vi "ClientForSingleDeviceDServer_01.vi"() -> ()   [LabVIEW 2014, in "examples.lvlib"]
uses:
  vis/tango_vi.llb/avToShortImage.vi
  vis/tango_vi.llb/avToLongSpectrum.vi
  vis/tango_vi.llb/avToDoubleScalar.vi
  vis/tango_vi.llb/avToStringScalarAv.vi
  examples.lvlib
  vis/tango_vi.llb/tango.lvlib
panel:
  out "timestamp":string
  out "?":string
  out "attribute name":string
  out "quality":string
  out "?":i16[][](graph)
  out "value":dbl(graph)
  out "?":i32[](graph)
  out "success":bool=TRUE
  in  "<TangoTest> device name":string="labview/device/1"
  in  "Attribute names":string[](array[string])=["devDoubleScalar", "devLongSpectrum", "devShortImage", "devStringScalar"]
  # "TANGO  Binding for LabVIEW - LabVIEW DServer Client Example"
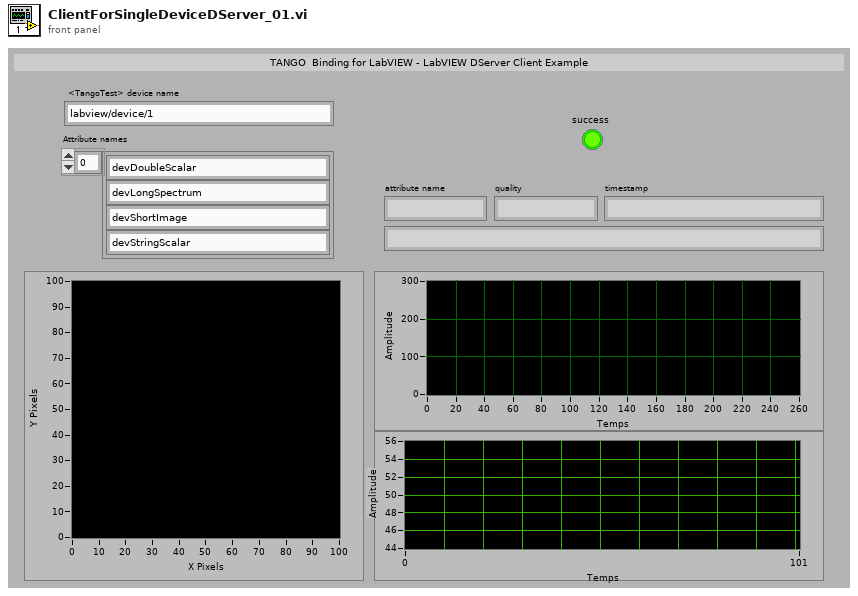
[diagram p1: front panel]
types:
  T1 = typedef "tango.lvlib/_AttributeValue_t.ctl" = cluster{"device name":string, "attribute name":string, "quality value":T2, "quality string":string, "timestamp":dbl, "dim. x":i32, "dim. y":i32, "value":u8[], "error code":i32, "error stack":string[], "data type":T3}
  T2 = typedef "tango.lvlib/_AttributeQuality_t.ctl" = enum16{"VALID", "INVALID", "ALARM", "CHANGING", "UNKNOWN_QUALITY"}
  T3 = typedef "tango.lvlib/_AttributeDataType_t.ctl" = enum16{"STATE_SCA", "STATE_SPE", "STATE_IMG", "STRING_SCA", "STRING_SPE", "STRING_IMG", "BOOL_SCA", "BOOL_SPE", "BOOL_IMG", "UCHAR_SCA", "UCHAR_SPE", "UCHAR_IMG", "SHORT_SCA", "SHORT_SPE", "SHORT_IMG", "USHORT_SCA", "USHORT_SPE", "USHORT_IMG", "LONG_SCA", "LONG_SPE", "LONG_IMG", "ULONG_SCA", "ULONG_SPE", "ULONG_IMG", "LONG64_SCA", "LONG64_SPE", "LONG64_IMG", "ULONG64_SCA", "ULONG64_SPE", "ULONG64_IMG", "FLOAT_SCA", "FLOAT_SPE", "FLOAT_IMG", "DOUBLE_SCA", "DOUBLE_SPE", "DOUBLE_IMG", "ENUM_SCA", "UNKNOWN_DATA_TYPE"}
  T4 = cluster{"device name":string, "attribute name":string, "quality value":i16, "quality string":string, "timestamp":dbl, "dim. x":i32, "dim. y":i32, "value_out":string, "setpoint":string, "error code":i32, "error stack":string[], "data type":u16}
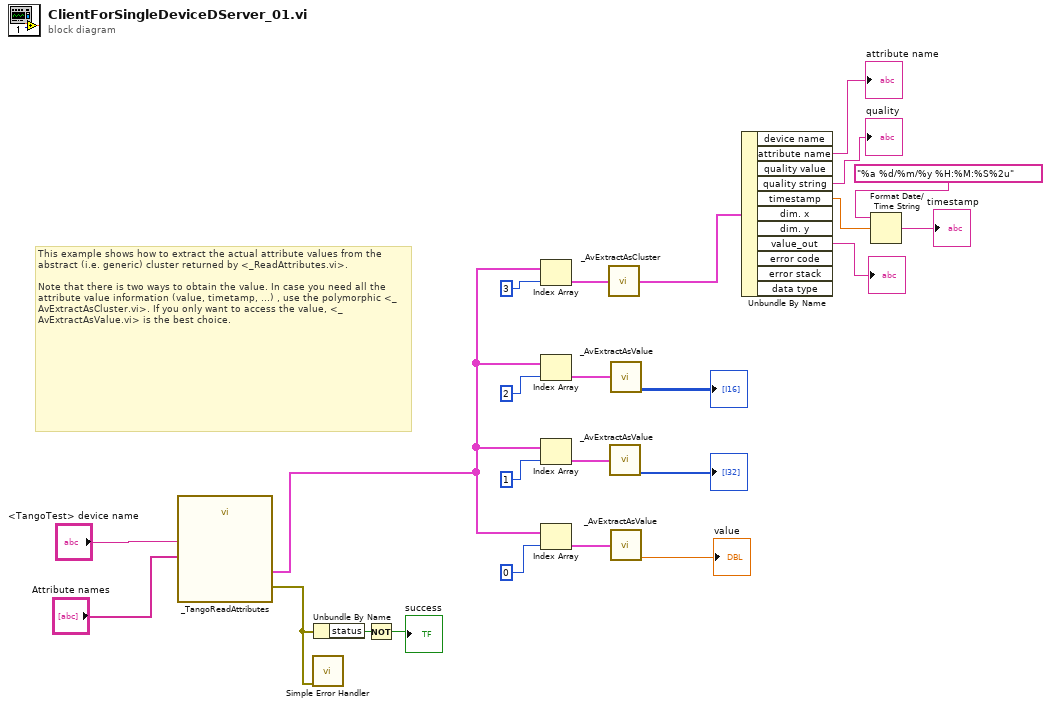
[diagram p0: block diagram]
diagram:
  # "This example shows how to extract the actual attribute values from the abstract (i.e. generic) cluster returned by <_ReadAttributes.vi>. \n\nNote that there is two ways to obtain the value. In case you need all the attribute value information (value, timetamp, ...) , use the polymorphic <_AvExtractAsCluster.vi>. If you only want to access the value, <_AvExtractAsValue.vi> is the best choice."
  n1 = call "_TangoReadAttributes.vi"("attribute names"="Attribute names", "device name"="<TangoTest> device name") -> ("error out"=w2:errorcluster, "attribute values"=w24:T1[])  [unwired: 1 in]
  n2 = call <vilib>:"Simple Error Handler.vi"("error in (no error)"=w2) -> ()  [unwired: 4 in, 5 out]
  n3 = Unbundle By Name(w2) -> ("status"=w3:bool)
  n4 = Not(x=w3) -> (.not. x?=→"success":bool)
  n5 = Index Array(array=w24, index=3 ("indice")) -> (element=w8:T1)
  n6 = Index Array(array=w24, index=2 ("indice")) -> (element=w7:T1)
  n7 = Index Array(array=w24, index=1 ("indice")) -> (element=w6:T1)
  n8 = Index Array(array=w24, index=0 ("indice")) -> (element=w5:T1)
  n9 = call-poly "_AvExtractAsCluster.vi"("attribute value"=w8) -> ("av"=w15:T4)
  n10 = call-poly "_AvExtractAsValue.vi"("attribute value"=w6) -> ("value"=→"?":i32[])  [unwired: 4 out]
  n11 = call-poly "_AvExtractAsValue.vi"("attribute value"=w7) -> ("value"=→"?":i16[][])  [unwired: 4 out]
  n12 = call-poly "_AvExtractAsValue.vi"("attribute value"=w5) -> ("value"=→"value":dbl)  [unwired: 4 out]
  n13 = Unbundle By Name(w15) -> ("attribute name"=→"attribute name":string, "quality string"=→"quality":string, "timestamp"=w14:dbl, "value_out"=→"?":string)  [unwired: 7 out]
  n14 = Format Date/Time String(time format string (%c)="%a %d/%m/%y %H:%M:%S%2u" ("chaîne de format de l'heure (%c)"), seconds (now)=w14) -> (date/time string=→"timestamp":string)  [unwired: 1 in]
